vi "AndorSeperateSif.vi"(8 "error in":errorcluster, 9 "Number":i32, 10 "Time":string="20170612", 11 "FilePath":string="C:\\Users\\light\\Desktop\\Andor\\data") -> (0 "error out":errorcluster, 3 "SaveStatus":bool)   [LabVIEW 2014]
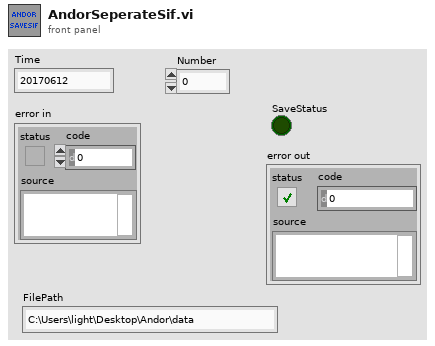
[diagram p1: front panel]
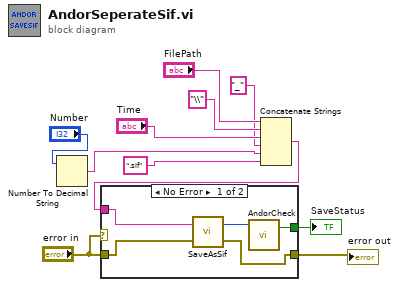
[diagram p0: block diagram]
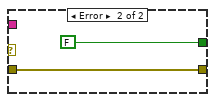
[diagram p2: hidden frame]
diagram:
  n1 = Number To Decimal String(number="Number") -> (decimal integer string=w1:string)  [unwired: 1 in]
  n2 = Concatenate Strings("FilePath", "\\" ("string"), "Time", "_" ("string"), w1, ".sif" ("string")) -> (w6:string)
  n3 = case shown="No Error" "error in" {
    tunnel: "error in" -> [w14 w17]
    tunnel: [w16 FALSE ("Status")] -> w10
    tunnel: [w12 w17] -> w9
    tunnel: w6 -> [w13 _]
    frame No Error {
      n4 = call <userlib>:"SaveAsSif.vi"("error in (no error)"=w14, "path"=w13) -> ("error out"=w12:errorcluster, "DLL error code"=w15:u32)
      n5 = call "AndorCheck.vi"("Input"=w15) -> ("Status"=w16:bool)  [unwired: 1 in, 1 out]
    }
    frame Error {
    }
  }
  "SaveStatus" <- w10
  "error out" <- w9
